vi "Update CPU Graph.vi"(8 "error in (no error)":errorcluster, 9 "df":dbl, 10 "Plot":sgl[](array[numeric]), 11 "Application Manager in":refnum<class "Application Manager.lvclass">) -> (0 "error out":errorcluster, 3 "Application Manager out":refnum<class "Application Manager.lvclass">)   [LabVIEW 2020, in "Application Manager.lvlib" / "Application Manager.lvclass"]
uses:
  Application Manager.lvclass
  <vilib>/ActorFramework/Message Enqueuer/Message Priority.ctl
  Application Manager.lvclass/Application Manager.ctl
  Simple UI/Simple UI Messages/Update CPU Graph Msg/Update CPU Graph Msg.lvclass/Update CPU Graph Msg.ctl
  <vilib>/ActorFramework/Message Enqueuer/Message Enqueuer.lvclass/Message Enqueuer.ctl
  <vilib>/ActorFramework/Message Enqueuer/Enqueue.vi
  Simple UI/Simple UI Messages/Update CPU Graph Msg/Update CPU Graph Msg.lvclass
  C:/Program Files/National Instruments/LabVIEW 2026/vi.lib/ActorFramework/Message/Message.lvclass
  <vilib>/ActorFramework/Message Priority Queue/Priority Enqueue.vi
  <vilib>/ActorFramework/Message Enqueuer/Message Enqueuer.lvclass
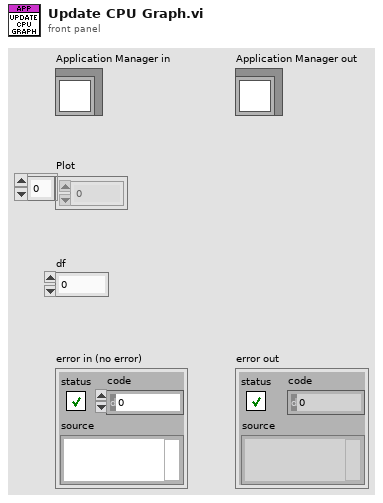
[diagram p1: front panel]
types:
  T1 = typedef "Actor Framework.lvlib/Message Enqueuer.lvclass/Message Priority.ctl" = enum16{"Low", "Normal", "High"}
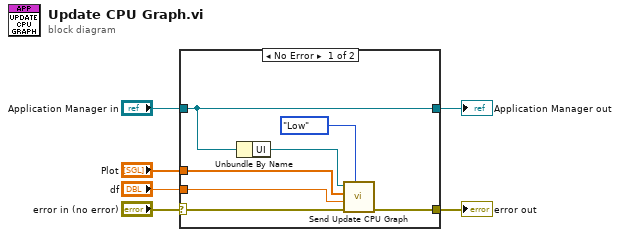
[diagram p0: block diagram]
diagram:
  n1 = case shown="No Error" "error in (no error)" {
    selector: "error in (no error)" -> [w13 w15]
    tunnel: [w10 w15] -> w5
    tunnel: [w9 w14] -> w3
    tunnel: "Application Manager in" -> [w9 w14]
    tunnel: "df" -> [w12 _]
    tunnel: "Plot" -> [w11 _]
    frame No Error {
      n2 = Unbundle By Name(w9) -> ("UI"=w8:refnum<class "Message Enqueuer.lvclass">)
      n3 = call "Send Update CPU Graph.vi"("Message Priority (Normal)"=Message_Priority."Low", "error in (no error)"=w13, "df"=w12, "Plot"=w11, "Message Enqueuer"=w8) -> ("error out"=w10:errorcluster)  [unwired: 5 in, 1 out]
    }
    frame Error {
    }
  }
  "error out" <- w5
  "Application Manager out" <- w3
